vi "Calculate conductance ITX_R and Theta.vi"(9 "index":T2={"N1"=1, "N2"=2, "N3"=3, "N4"=4, "V1_X"=4, "V1_Y"=5, "V2_X"=14, "V2_Y"=15, "CURRENT_X"=6, "Vsg"=1, "CURRENT_Y"=7}, 10 "File or Folder Path":path=path "C:/Users/ansom/Google Drive/ansom/Data/MNK/SA03018H.20170516/5 - sweep B, Vsg lockin") -> (0 "N Array":T1(array[cluster])=[{"N1"=-0.14999999999999997, "N2"=27.266186760598742, "N3"=-17.8854, "N4"=0.0001000063641536694}, {"N1"=-0.14999999999999997, "N2"=26.846695511611152, "N3"=-17.6639, "N4"=9.9910078820074e-05}, {"N1"=-0.14999999999999997, "N2"=26.644619458735516, "N3"=-17.4419, "N4"=0.00010001461278028781}, {"N1"=-0.14999999999999997, "N2"=26.394910452509276, "N3"=-17.2204, "N4"=0.00010017377349041838}, {"N1"=-0.14999999999999997, "N2"=26.17876966960713, "N3"=-16.9989, "N4"=0.00010004441930687711}, {"N1"=-0.14999999999999997, "N2"=25.918232519878988, "N3"=-16.7768, "N4"=0.00010016176496881128}, {"N1"=-0.14999999999999997, "N2"=25.799962248117083, "N3"=-16.5555, "N4"=9.984181147148092e-05}, {"N1"=-0.14999999999999997, "N2"=25.67213314559327, "N3"=-16.3341, "N4"=0.00010025789749806366}, {"N1"=-0.14999999999999997, "N2"=25.562395299716517, "N3"=-16.1123, "N4"=9.989344508808523e-05}, {"N1"=-0.14999999999999997, "N2"=25.43779166285741, "N3"=-15.8915, "N4"=9.981914917166688e-05}, {"N1"=-0.14999999999999997, "N2"=25.35387471065981, "N3"=-15.669, "N4"=9.997972760482823e-05}, {"N1"=-0.14999999999999997, "N2"=25.311318320839742, "N3"=-15.4483, "N4"=0.00010004234444651203}], 8 "angle theta":dbl[](array[numeric]), 11 "Resistance/Conductance vs Vsg":cluster{dbl[], dbl[]}[](graph))   [LabVIEW 2016]
uses:
  <vilib>/Utility/miscctls.llb/LVOffsetAndMultiplierTypeDef.ctl
  <vilib>/Analysis/2dsp.llb/Decimate (single shot, DBL).vi
  <vilib>/Analysis/3filter.llb/Savitzky-Golay Filter (DBL).vi
  <userlib>/LevyLab/LV to ITX/LVtoITX.lvclass
  <vilib>/Analysis/NI_AALBase.lvlib
  <vilib>/Analysis/NI_AALPro.lvlib
panel:
  in  "e^2/h?":bool=TRUE
  in  "A offset 2":dbl format="%#_6p"
  in  "Ring":u16(ring) items=["default", "DIFF"]
  in  "Portion of data":cluster{dbl, dbl}(slide)={0.75, 0.25} scale=0.0..1.0
  in  "dy/dx vs x":bool=TRUE
  in  "fit points":dbl=10.0
  in  "side points":i32=6
  in  "decimating factor":i32=1
  in  "length 2":i32=1000
  in  "index 2":i32
  in  "T=conductance\nF=resistance":bool=TRUE
  in  "log scale?":bool
  in  "calculate Ey":bool
  out "E 2":dbl[][](graph)
  out "counter":i32=11
  out "Path":path=path "C:/Users/ansom/Google Drive/ansom/Data/MNK/SA03018H.20170516/5 - sweep B, Vsg lockin/SA03018H.20170516.000011.itx"
  out "Comments":string="IGOR\nX// Date: 5/18/2017 2:21 PM\nX// B = -18 T to 18 T, 0.03 T/min\nX// sweep Vsg: -150mV to 300mV, 1mV steps\nX// axis1: 167\nX// axis 2=261\nX// Vbg=-6.58V\nX// \nX// lockin:\nX// 0: 2, voltage, V+\nX// 1: 3, current, 100uV AC, 175uV DC, 13 Hz\nX// 2: 4, voltage, V+\nX// 3: 5, n.c.\nX// 4: 7, current, drain\nX// 5: 28, voltage V-\nX// \nX// KH gain=100x, shunt resistor=50kOhm\n\n\n\n\n\n\n\n\n\n\n\n\n\n\n\n\n\n\n\n\n\n\n\n\n\n\n\n\n\n\n\n\n\n\n\n\n\n\n\n\n\n\nX \nX Display/R 'time.SA03018H.20170516.000011'\nX AppendToGraph 'Vsg.SA03018H.20170516.000011'\nX AppendToGraph 'T.SA03018H.20170516.000011'\nX AppendToGraph 'B.SA03018H.20170516.000011'\nX AppendToGraph 'X0.SA03018H.20170516.000011'\nX AppendToGraph 'Y0.SA03018H.20170516.000011'\nX AppendToGraph 'X1.SA03018H.20170516.000011'\nX AppendToGraph 'Y1.SA03018H.20170516.000011'\nX AppendToGraph 'X2.SA03018H.20170516.000011'\nX AppendToGraph 'Y2.SA03018H.20170516.000011'\nX AppendToGraph 'X3.SA03018H.20170516.000011'\nX AppendToGraph 'Y3.SA03018H.20170516.000011'\nX AppendToGraph 'X4.SA03018H.20170516.000011'\nX AppendToGraph 'Y4.SA03018H.20170516.000011'\nX AppendToGraph 'X5.SA03018H.20170516.000011'\nX AppendToGraph 'Y5.SA03018H.20170516.000011'\nX AppendToGraph 'B_rate.SA03018H.20170516.000011'\nX AppendToGraph 'R4t(e2/h).SA03018H.20170516.000011'\nX AppendToGraph 'axis1.SA03018H.20170516.000011'\nX AppendToGraph 'axis2.SA03018H.20170516.000011'\nX Label bottom \"x label\"\nX Label left \"y label\"\nX ModifyGraph rgb('time.SA03018H.20170516.000011')=(65280,0,0)\nX ModifyGraph rgb('Vsg.SA03018H.20170516.000011')=(65280,18432,0)\nX ModifyGraph rgb('T.SA03018H.20170516.000011')=(65280,35328,0)\nX ModifyGraph rgb('B.SA03018H.20170516.000011')=(65280,52224,0)\nX ModifyGraph rgb('X0.SA03018H.20170516.000011')=(60416,65280,0)\nX ModifyGraph rgb('Y0.SA03018H.20170516.000011')=(41984,65280,0)\nX ModifyGraph rgb('X1.SA03018H.20170516.000011')=(25088,65280,0)\nX ModifyGraph rgb('Y1.SA03018H.20170516.000011')=(8192,65280,0)\nX ModifyGraph rgb('X2.SA03018H.20170516.000011')=(0,65280,10240)\nX ModifyGraph rgb('Y2.SA03018H.20170516.000011')=(0,65280,28672)\nX ModifyGraph rgb('X3.SA03018H.20170516.000011')=(0,65280,45568)\nX ModifyGraph rgb('Y3.SA03018H.20170516.000011')=(0,65280,62464)\nX ModifyGraph rgb('X4.SA03018H.20170516.000011')=(0,50176,65280)\nX ModifyGraph rgb('Y4.SA03018H.20170516.000011')=(0,31744,65280)\nX ModifyGraph rgb('X5.SA03018H.20170516.000011')=(0,14848,65280)\nX ModifyGraph rgb('Y5.SA03018H.20170516.000011')=(2048,0,65280)\nX ModifyGraph rgb('B_rate.SA03018H.20170516.000011')=(20480,0,65280)\nX ModifyGraph rgb('R4t(e2/h).SA03018H.20170516.000011')=(38912,0,65280)\nX ModifyGraph rgb('axis1.SA03018H.20170516.000011')=(55808,0,65280)\nX ModifyGraph rgb('axis2.SA03018H.20170516.000011')=(65280,0,58368)\nX Legend/C/N=text0/J \"\\\\s('time.SA03018H.20170516.000011') time\\r\\\\s('Vsg.SA03018H.20170516.000011') Vsg\\r\\\\s('T.SA03018H.20170516.000011') T\\r\\\\s('B.SA03018H.20170516.000011') B\\r\\\\s('X0.SA03018H.20170516.000011') X0\\r\\\\s('Y0.SA03018H.20170516.000011') Y0\\r\\\\s('X1.SA03018H.20170516.000011') X1\\r\\\\s('Y1.SA03018H.20170516.000011') Y1\\r\\\\s('X2.SA03018H.20170516.000011') X2\\r\\\\s('Y2.SA03018H.20170516.000011') Y2\\r\\\\s('X3.SA03018H.20170516.000011') X3\\r\\\\s('Y3.SA03018H.20170516.000011') Y3\\r\\\\s('X4.SA03018H.20170516.000011') X4\\r\\\\s('Y4.SA03018H.20170516.000011') Y4\\r\\\\s('X5.SA03018H.20170516.000011') X5\\r\\\\s('Y5.SA03018H.20170516.000011') Y5\\r\\\\s('B_rate.SA03018H.20170516.000011') B_rate\\r\\\\s('R4t(e2/h).SA03018H.20170516.000011') R4t (e2/h)\\r\\\\s('axis1.SA03018H.20170516.000011') axis 1\\r\\\\s('axis2.SA03018H.20170516.000011') axis 2\"\nX ModifyGraph mirror(bottom)=1\nX ModifyGraph width=216\nX ModifyGraph height={Aspect,0.6}\nX ModifyGraph Log(bottom)=0\nX ModifyGraph Log(left)=0\nX \n"
  in  "file contains 2D data?":bool
  out "Index, Wavenames":string[][](table)=[["0", "'time.SA03018H.20170516.000011'\n"], ["1", "'Vsg.SA03018H.20170516.000011'\n"], ["2", "'T.SA03018H.20170516.000011'\n"], ["3", "'B.SA03018H.20170516.000011'\n"], ["4", "'X0.SA03018H.20170516.000011'\n"], ["5", "'Y0.SA03018H.20170516.000011'\n"], ["6", "'X1.SA03018H.20170516.000011'\n"], ["7", "'Y1.SA03018H.20170516.000011'\n"], ["8", "'X2.SA03018H.20170516.000011'\n"], ["9", "'Y2.SA03018H.20170516.000011'\n"], ["10", "'X3.SA03018H.20170516.000011'\n"], ["11", "'Y3.SA03018H.20170516.000011'\n"], ["12", "'X4.SA03018H.20170516.000011'\n"], ["13", "'Y4.SA03018H.20170516.000011'\n"], ["14", "'X5.SA03018H.20170516.000011'\n"], ["15", "'Y5.SA03018H.20170516.000011'\n"], ["16", "'B_rate.SA03018H.20170516.000011'\n"], ["17", "'R4t(e2/h).SA03018H.20170516.000011'\n"], ["18", "'axis1.SA03018H.20170516.000011'\n"], ["19", "'axis2.SA03018H.20170516.000011'\n"], ["", ""]]
  out "N":cluster{"N1":dbl, "N2":dbl, "N3":dbl, "N4":dbl}={"N1"=-0.14999999999999997, "N2"=25.311318320839742, "N3"=-15.4483, "N4"=0.00010004234444651203} {"N4" format="%#_6p"; "N3" format="%#_6p"; "N2" format="%#_6p"; "N1" format="%#_6p"}
  in  "Ey":T3={"Offset"=0.0, "Multiplier"=1.0}
  in  "Ex":T3={"Offset"=0.0, "Multiplier"=1.0}
  in  "recolor traces?":bool
  out "Theta vs Vsg":cluster{dbl[], dbl[]}[](graph)
  out "E":dbl[][](graph)
  in  "B x name":string="Vsg (V)"
  in  "A y name":string="Conductance (S)"
  in  "Ex name":string="Ex name"
  in  "Ez name":string="Ez name"
  in  "D x name":string="Vsg (V)"
  in  "C y name":string="Conductance (S)"
  in  "Ey name":string="Ey name"
  out "time":string[][](table)=[["5/18/2017", "1:00 PM"], ["5/18/2017", "1:07 PM"], ["5/18/2017", "1:15 PM"], ["5/18/2017", "1:22 PM"], ["5/18/2017", "1:29 PM"], ["5/18/2017", "1:37 PM"], ["5/18/2017", "1:44 PM"], ["5/18/2017", "1:52 PM"], ["5/18/2017", "1:59 PM"], ["5/18/2017", "2:07 PM"], ["5/18/2017", "2:14 PM"], ["5/18/2017", "2:21 PM"]]
  in  "offset":i32
  in  "length":i32=1000
  in  "B is time?":bool
  in  "D  is time?":bool
  in  "Generate Folder Index File?":bool
  in  "pattern":string="*.itx"
  in  "Use Folder Index File?":bool
  # "CURRENT/(V1-V2)"
  # "CURRENT/(V3-V4)"
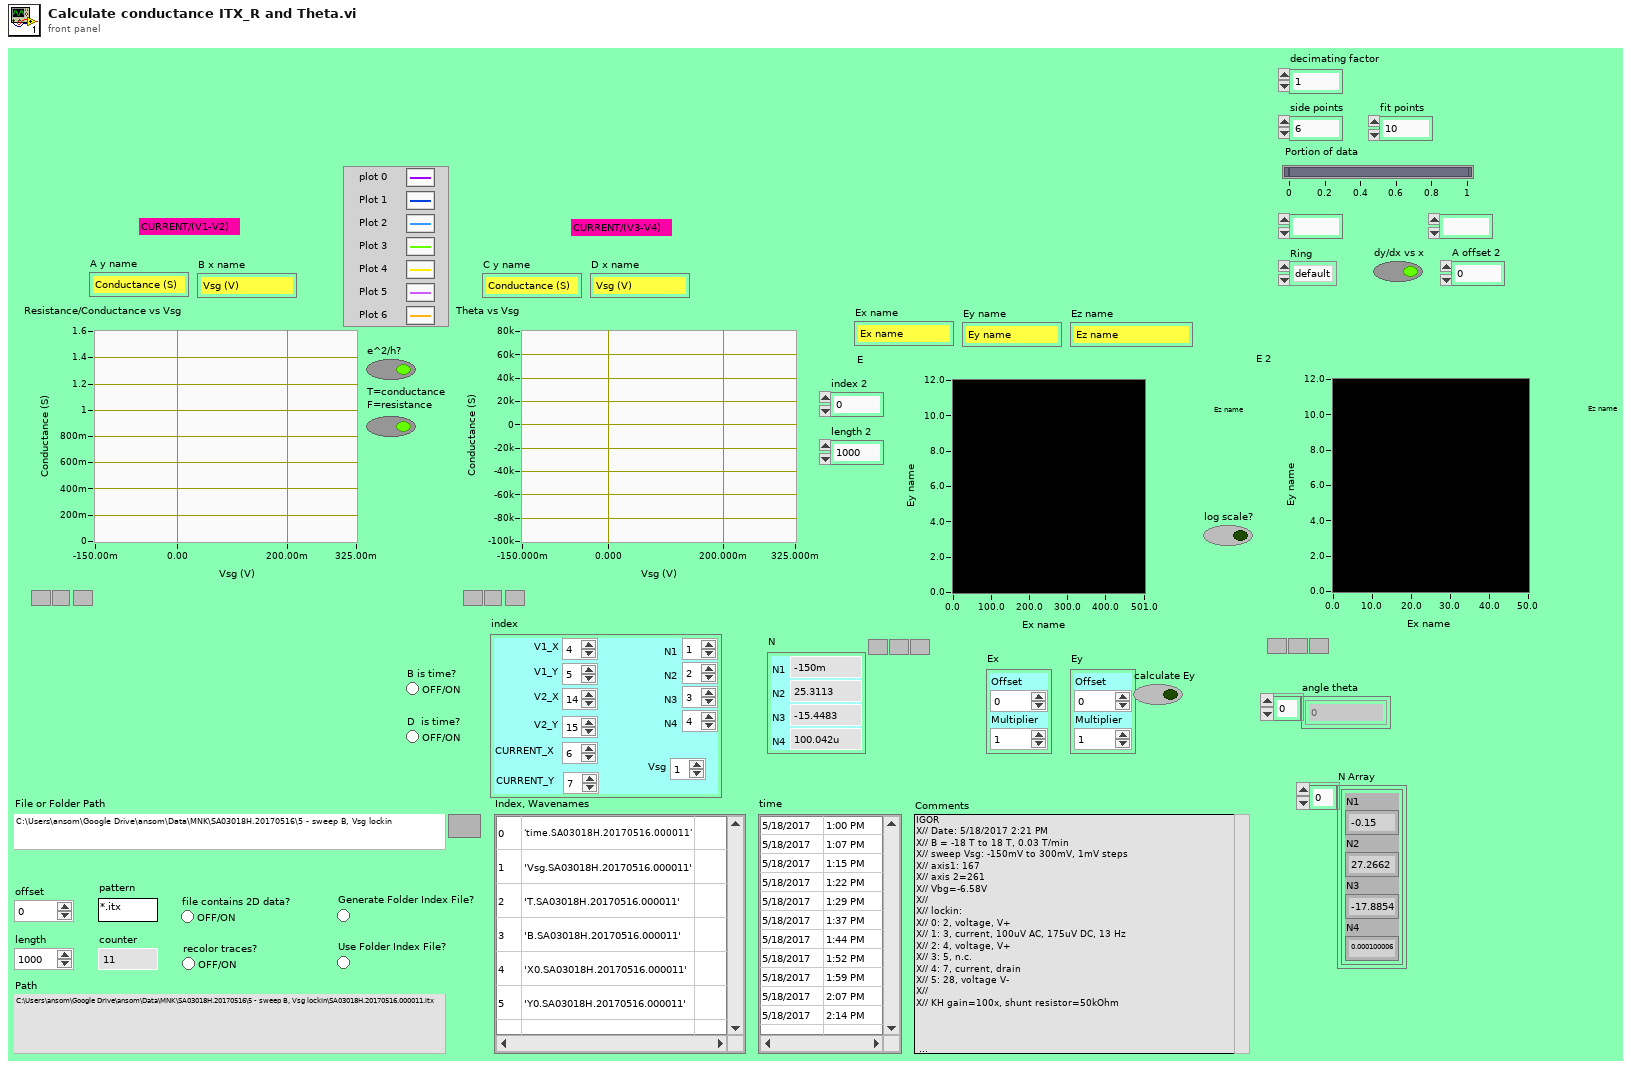
[diagram p1: front panel]
types:
  T1 = cluster{"N1":dbl, "N2":dbl, "N3":dbl, "N4":dbl}[]
  T2 = cluster{"N1":i32, "N2":i32, "N3":i32, "N4":i32, "V1_X":i32, "V1_Y":i32, "V2_X":i32, "V2_Y":i32, "CURRENT_X":i32, "Vsg":i32, "CURRENT_Y":i32}
  T3 = typedef "LVOffsetAndMultiplierTypeDef.ctl" = cluster{"Offset":dbl, "Multiplier":dbl}
  T4 = cluster{"Decimated Array":dbl[], "Decimated Array":dbl[]}
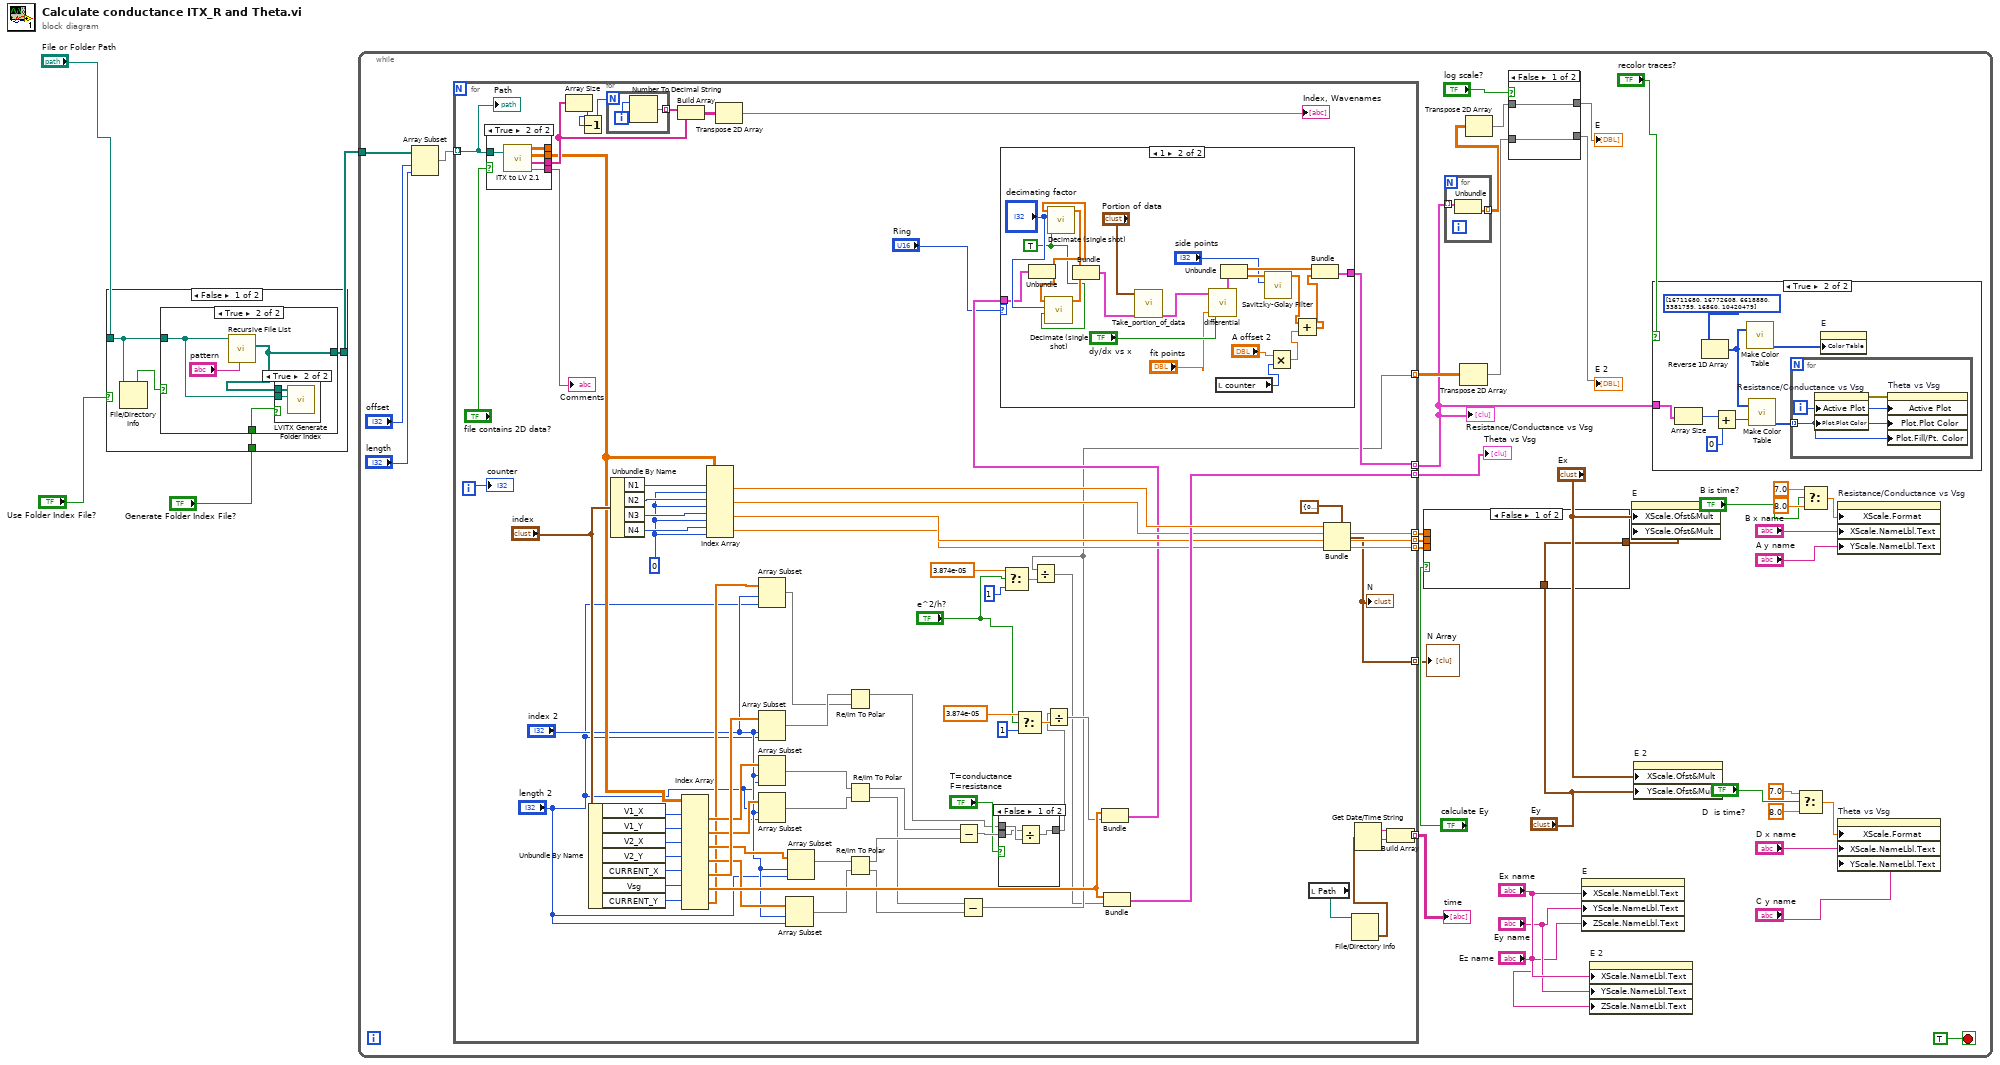
[diagram p0: block diagram]
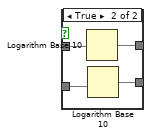
[diagram p2: hidden frame]
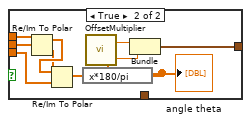
[diagram p3: hidden frame]
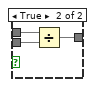
[diagram p6: hidden frame]
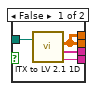
[diagram p7: hidden frame]
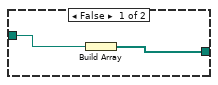
[diagram p8: hidden frame]
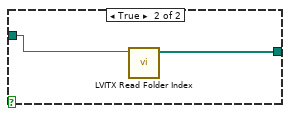
[diagram p10: hidden frame]
diagram:
  n1 = case shown="False" "Use Folder Index File?" {
    tunnel: [w6 w17] -> w2
    tunnel: "File or Folder Path" -> [w8 w18]
    tunnel: "Generate Folder Index File?" -> [w5 _]
    frame False {
      n2 = File/Directory Info(path=w8) -> (directory=w7:bool)  [unwired: 1 in, 6 out]
      n3 = case shown="True" w7 {
        tunnel: [w10 w13] -> w6
        tunnel: w8 -> [w9 w12]
        tunnel: w5 -> [_ w11]
        frame False {
          n4 = Build Array(w9) -> (w10:path[])
        }
        frame True {
          n5 = call <vilib>:"Recursive File List.vi"("pattern"="pattern", "Folder Path"=w12) -> ("All Files in Dir"=w13:path[])  [unwired: 5 in, 4 out]
          n6 = case shown="True" w11 {
            tunnel: w13 -> [_ w16]
            tunnel: w12 -> [_ w15]
            frame False {
            }
            frame True {
              n7 = call <userlib>:"LVITX Generate Folder Index.vi"("File or Folder Path"=w15, "All Files in Dir"=w16) -> ()  [unwired: 10 in]
            }
          }
        }
      }
    }
    frame True {
      n8 = call <userlib>:"LVITX Read Folder Index.vi"("File or Folder Path"=w18) -> ("Array"=w17:path[])  [unwired: 10 in]
    }
  }
  n9 = while {
    tunnel: w2 -> [w49]
    stop <- TRUE stop-if-true
    n10 = Array Subset(array=w49, index="offset", length="length") -> (w48:path[])
    n11 = for {
      tunnel: w48 -> [w157] mode=indexing
      tunnel: [w157] -> _ mode=indexing
      tunnel: [w139] -> w52 mode=indexing
      tunnel: [w100] -> w21 mode=indexing
      tunnel: [w129] -> w39 mode=indexing
      tunnel: [w90] -> w38 mode=indexing
      tunnel: [w125] -> w32 mode=indexing
      tunnel: [w124] -> w31 mode=indexing
      tunnel: [w123] -> w30 mode=indexing
      tunnel: [w87] -> w19 mode=indexing
      i -> [w126]
      w137 = 0 ("disabled index (col)")
      n12 = case shown="True" "file contains 2D data?" {
        tunnel: [w193 w196] -> w158
        tunnel: [w191 w197] -> w132
        tunnel: w157 -> [w192 w198]
        tunnel: [w190 w195] -> w150
        tunnel: [w191 w194] -> _
        frame False {
          n13 = call <userlib>:"ITX to LV 2.1 1D.vi"("file (use dialog)"=w192) -> ("array type (2D Dbl)"=w191:dbl[][], "wave names"=w190:string[], "Notes"=w193:string)  [unwired: 2 in]
        }
        frame True {
          n14 = call <userlib>:"ITX to LV 2.1.vi"("file (use dialog)"=w198) -> ("2D array"=w194:dbl[][], "1D arrays"=w197:dbl[][], "wave names"=w195:string[], "Notes"=w196:string)  [unwired: 1 in]
        }
      }
      "Comments" <- w158
      n15 = Array Size(array=w150) -> (size(s)=w153:i32)
      n16 = Decrement(x=w153) -> (x-1=w152:i32)
      n17 = Unbundle By Name("index") -> ("V1_X"=w136:i32, "V1_Y"=w135:i32, "V2_X"=w134:i32, "V2_Y"=w133:i32, "CURRENT_X"=w131:i32, "Vsg"=w128:i32, "CURRENT_Y"=w108:i32)
      n18 = for {
        N: w152 -> [_]
        tunnel: [w188] -> w155 mode=indexing
        i -> [w189]
        n19 = Number To Decimal String(number=w189) -> (decimal integer string=w188:string)  [unwired: 1 in]
      }
      n20 = Unbundle By Name("index") -> ("N1"=w145:i32, "N2"=w146:i32, "N3"=w147:i32, "N4"=w148:i32)
      n21 = Build Array(w155, w150) -> (w151:string[][])
      n22 = Index Array(array=w132, index (row) #1=w136, index (row) #2=w135, index (row) #3=w134, index (row) #4=w133, index (row) #5=w131, index (row) #6=w128, index (row) #7=w108) -> (element #1=w120:dbl[], element #2=w119:dbl[], element #3=w118:dbl[], element #4=w117:dbl[], element #5=w121:dbl[], element #6=w127:dbl[], element #7=w107:dbl[])  [unwired: 7 in]
      n23 = Index Array(array=w132, index (row) #1=w145, index (col) #1=w137, index (row) #2=w146, index (col) #2=w137, index (row) #3=w147, index (col) #3=w137, index (row) #4=w148, index (col) #4=w137) -> (element #1=w143:dbl, element #2=w125:dbl, element #3=w124:dbl, element #4=w123:dbl)
      n24 = Transpose 2D Array(2D array=w151) -> (transposed array=→"Index, Wavenames":string[][])
      n25 = Array Subset(array=w107, index="index 2", length="length 2") -> (w103:dbl[])
      n26 = Array Subset(array=w121, index="index 2", length="length 2") -> (w104:dbl[])
      n27 = Array Subset(array=w120, index="index 2", length="length 2") -> (w116:dbl[])
      n28 = Array Subset(array=w119, index="index 2", length="length 2") -> (w115:dbl[])
      n29 = Array Subset(array=w117, index="index 2", length="length 2") -> (w112:dbl[])
      n30 = Array Subset(array=w118, index="index 2", length="length 2") -> (w113:dbl[])
      n31 = Re/Im To Polar(2:w103, 3:w104) -> (1:w102:dbl[])  [unwired: 1 out]
      n32 = Re/Im To Polar(2:w115, 3:w116) -> (0:w110:dbl[], 1:w114:dbl[])
      n33 = Re/Im To Polar(2:w112, 3:w113) -> (0:w109:dbl[], 1:w111:dbl[])
      n34 = Subtract(x=w114, y=w111) -> (x-y=w130:dbl[])
      n35 = Subtract(x=w110, y=w109) -> (x-y=w90:dbl[])
      n36 = case shown="False" "T=conductance\nF=resistance" {
        tunnel: w130 -> [w182 w187]
        tunnel: w102 -> [w183 w186]
        tunnel: [w184 w185] -> w88
        frame False {
          n37 = Divide(x=w182, y=w183) -> (x/y=w184:dbl[])
        }
        frame True {
          n38 = Divide(x=w186, y=w187) -> (x/y=w185:dbl[])
        }
      }
      n39 = Select(t=3.874e-05, s="e^2/h?", f=1) -> (s? t:f=w95:dbl)
      n40 = Select(t=3.874e-05, s="e^2/h?", f=1) -> (s? t:f=w96:dbl)
      n41 = Divide(x=w90, y=w95) -> (x/y=w89:dbl[])
      n42 = Divide(x=w88, y=w96) -> (x/y=w92:dbl[])
      n43 = Bundle("1D arrays"=w127, w92) -> (w101:cluster{"1D arrays":dbl[], dbl[]})  [unwired: 1 in]
      n44 = case shown="1" "Ring" {
        tunnel: w101 -> [w159 w165]
        tunnel: [w159 w174] -> w100
        frame 0, Default {
        }
        frame 1 {
          w166 = TRUE ("averaging")
          n45 = Unbundle(w165) -> ("1D arrays"=w171:dbl[], w169:dbl[])
          n46 = call-poly <vilib>:"Decimate (single shot).vi"("averaging"=w166, "decimating factor"="decimating factor", "X"=w169) -> ("Decimated Array"=w168:dbl[])  [unwired: 7 in, 1 out]
          n47 = call-poly <vilib>:"Decimate (single shot).vi"("averaging"=w166, "decimating factor"="decimating factor", "X"=w171) -> ("Decimated Array"=w170:dbl[])  [unwired: 7 in, 1 out]
          n48 = Bundle("Decimated Array"=w170, "Decimated Array"=w168) -> (w172:T4)  [unwired: 1 in]
          n49 = call <userlib>:"Take_portion_of_data.vi"("input IV"=w172, "Slide"="Portion of data") -> ("Output IV"=w179:cluster{dbl[], dbl[]})  [unwired: 5 in]
          n50 = call <userlib>:"differential.vi"("Numeric"="fit points", "dy/dx vs x"="dy/dx vs x", "A vs B 2"=w179) -> ("A vs B 3"=w175:T4)  [unwired: 1 in]
          n51 = local read "counter"() -> (w161:i32)
          n52 = Unbundle(w175) -> ("Decimated Array"=w177:dbl[], "Decimated Array"=w176:dbl[])
          n53 = call-poly <vilib>:"Savitzky-Golay Filter.vi"("side points"="side points", "X"=w176) -> ("Filtered X"=w164:dbl[])  [unwired: 8 in, 1 out]
          n54 = Multiply(x="A offset 2", y=w161) -> (x*y=w160:dbl)
          n55 = Add(x=w164, y=w160) -> (x+y=w163:dbl[])
          n56 = Bundle("Decimated Array"=w177, w163) -> (w174:cluster{"Decimated Array":dbl[], dbl[]})  [unwired: 1 in]
        }
      }
      n57 = Bundle("1D arrays"=w127, w89) -> (w129:cluster{"1D arrays":dbl[], dbl[]})  [unwired: 1 in]
      n58 = local read "Path"() -> (w144:path)
      n59 = Bundle(cluster=cluster{"N1":dbl, "N2":dbl, "N3":dbl, "N4":dbl} {"N1"=0.0, "N2"=0.0, "N3"=0.0, "N4"=0.0}, "N1"=w143, "N2"=w125, "N3"=w124, "N4"=w123) -> (w87:cluster{"N1":dbl, "N2":dbl, "N3":dbl, "N4":dbl})
      "N" <- w87
      n60 = File/Directory Info(path=w144) -> (last mod=w142:timestamp)  [unwired: 1 in, 6 out]
      n61 = Get Date/Time String(seconds (now)=w142) -> (date string=w141:string, time string=w140:string)  [unwired: 2 in]
      n62 = Build Array(w141, w140) -> (w139:string[])
      "counter" <- w126
      "Path" <- w157
    }
    "Resistance/Conductance vs Vsg" <- w21
    "Theta vs Vsg" <- w39
    "time" <- w52
    "N Array" <- w19
    n63 = case shown="False" "calculate Ey" {
      tunnel: w32 -> [_ w75]
      tunnel: w31 -> [_ w74]
      tunnel: w30 -> [_ w72]
      tunnel: [w66 w68] -> w29
      tunnel: "Ey" -> [w66 _]
      frame False {
      }
      frame True {
        n64 = Re/Im To Polar(2:w74, 3:w75) -> (0:w71:dbl[], 1:w73:dbl[])
        n65 = Re/Im To Polar(2:w72, 3:w73) -> ()  [unwired: 2 out]
        n66 = expression code="x*180/pi"(w71) -> (w67:dbl[])
        "angle theta" <- w67
        n67 = call <userlib>:"OffsetMultiplier.vi"("Array"=w67) -> ("Offset"=w70:dbl, "Multiplier"=w69:dbl)
        n68 = Bundle("Offset"=w70, "Multiplier"=w69) -> (w68:cluster{"Offset":dbl, "Multiplier":dbl})  [unwired: 1 in]
      }
    }
    n69 = for {
      tunnel: w21 -> [w59] mode=indexing
      tunnel: [w58] -> w20 mode=indexing
      n70 = Unbundle(w59) -> (w58:dbl[])  [unwired: 1 out]
    }
    n71 = Transpose 2D Array(2D array=w38) -> (transposed array=w23:dbl[][])
    n72 = Transpose 2D Array(2D array=w20) -> (transposed array=w25:dbl[][])
    n73 = case shown="False" "log scale?" {
      tunnel: w25 -> [w61 w65]
      tunnel: [w61 w64] -> w24
      tunnel: w23 -> [w60 w63]
      tunnel: [w60 w62] -> w22
      frame False {
      }
      frame True {
        n74 = Logarithm Base 10(1:w65) -> (0:w64:dbl[][])
        n75 = Logarithm Base 10(1:w63) -> (0:w62:dbl[][])
      }
    }
    "E" <- w24
    "E 2" <- w22
    n76 = property on="E" class="IntGraph (strict)"("XScale.NameLbl.Text"="Ex name", "YScale.NameLbl.Text"="Ey name", "ZScale.NameLbl.Text"="Ez name") -> ()  [unwired: 2 in, 2 out]
    n77 = property on="E 2" class="IntGraph (strict)"("XScale.NameLbl.Text"="Ex name", "YScale.NameLbl.Text"="Ey name", "ZScale.NameLbl.Text"="Ez name") -> ()  [unwired: 2 in, 2 out]
    n78 = property on="E" class="IntGraph (strict)"("XScale.Ofst&Mult"="Ex", "YScale.Ofst&Mult"=w29) -> ()  [unwired: 2 in, 2 out]
    n79 = property on="E 2" class="IntGraph (strict)"("XScale.Ofst&Mult"="Ex", "YScale.Ofst&Mult"="Ey") -> ()  [unwired: 2 in, 2 out]
    n80 = case shown="True" "recolor traces?" {
      tunnel: w21 -> [_ w76]
      frame False {
      }
      frame True {
        n81 = Array Size(array=w76) -> (size(s)=w79:i32)
        n82 = Reverse 1D Array(array=u32[] [16711680, 16772608, 6618880, 3381759, 16860, 10420479] ("color scale")) -> (reversed array=w78:u32[])
        n83 = Add(x=w79, y=0 ("x")) -> (x+y=w83:i32)
        n84 = call <userlib>:"Make Color Table.vi"("Array"=w78) -> ("Color Tbl"=w81:u32[])  [unwired: 1 in, 3 out]
        n85 = call <userlib>:"Make Color Table.vi"("Array"=w78, "Size/3"=w83) -> ("Color Tbl"=w80:u32[])  [unwired: 3 out]
        n86 = for {
          tunnel: w80 -> [w84] mode=indexing
          i -> [w85]
          n87 = property on="Resistance/Conductance vs Vsg" class="XYGraph (strict)"("Active Plot"=w85, "Plot.Plot Color"=w84) -> (error out=w86:errorcluster)  [unwired: 2 in, 1 out]
          n88 = property on="Theta vs Vsg" class="XYGraph (strict)"(error in=w86, "Active Plot"=w85, "Plot.Plot Color"=w84, "Plot.Fill/Pt. Color"=w84) -> ()  [unwired: 1 in, 2 out]
        }
        n89 = property on="E" class="IntGraph (strict)"("Color Table"=w81) -> ()  [unwired: 2 in, 2 out]
      }
    }
    n90 = Select(t=7.0, s="D  is time?", f=8.0) -> (s? t:f=w44:dbl)
    n91 = Select(t=7.0, s="B is time?", f=8.0) -> (s? t:f=w45:dbl)
    n92 = property on="Resistance/Conductance vs Vsg" class="XYGraph (strict)"("XScale.Format"=w45, "XScale.NameLbl.Text"="B x name", "YScale.NameLbl.Text"="A y name") -> ()  [unwired: 2 in, 2 out]
    n93 = property on="Theta vs Vsg" class="XYGraph (strict)"("XScale.Format"=w44, "XScale.NameLbl.Text"="D x name", "YScale.NameLbl.Text"="C y name") -> ()  [unwired: 2 in, 2 out]
  }
